vi "Force reset UI controls.vi"(8 "error in (no error)":errorcluster) -> (0 "error out":errorcluster)   [LabVIEW 2017]
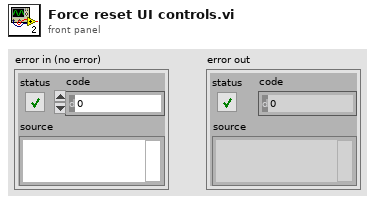
[diagram p1: front panel]
types:
  T1 = enum8{"Enabled", "Disabled", "Disabled and Grayed Out"}
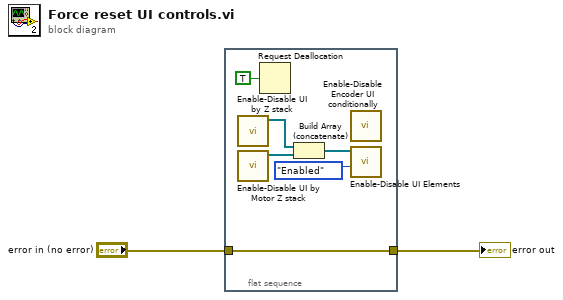
[diagram p0: block diagram]
diagram:
  n1 = flat-sequence {
    tunnel: "error in (no error)" -> [w3]
    tunnel: [w3] -> w1
    frame #0 {
      n2 = call "Enable-Disable UI by Z stack.vi"() -> ("Controls refs to enable/disable"=w6:refnum<vi>[])  [unwired: 11 in]
      n3 = call "Enable-Disable UI by Motor Z stack.vi"() -> ("Controls to disable"=w4:refnum<vi>[])  [unwired: 11 in]
      n4 = Request Deallocation(TRUE ("flag")) -> ()
      n5 = Build Array (concatenate)(w6, w4) -> (w5:refnum<vi>[])
      n6 = call "Enable-Disable Encoder UI conditionally.vi"() -> ()  [unwired: 11 in, 1 out]
      n7 = call "Enable-Disable UI Elements.vi"("Enable/Disable"=T1."Enabled", "Ctrl ref's"=w5) -> ()  [unwired: 9 in, 1 out]
    }
  }
  "error out" <- w1
